vi "Test Start.vi"(11 "Error in":errorcluster) -> (15 "Error out":errorcluster)   [LabVIEW 2020, in "StopWatchTests.lvlib"]
doc: "This VI is used for validating start button in stopwatch"
uses:
  StopWatchTests.lvlib
  <vilib>/SLL Drona/APIs/Stimulus/ControlValue/SetValueAuto.vi
  <vilib>/SLL Drona/APIs/Assert/AssertControlValue/Equal.vi
  <vilib>/SLL Drona/APIs/Get/GetControlValue/GetControlValueByPathString.vi
  <vilib>/SLL Drona/APIs/Stimulus/VI/CloseVI.vi
  <vilib>/Utility/error.llb/Error Cluster From Error Code.vi
  <vilib>/ErrorRing/Error Ring.xnode
  <vilib>/addons/_JKI Toolkits/Caraya/classes/Test/Test.lvclass
  <vilib>/SLL Drona/Drona.lvlib
  <vilib>/SLL Drona/APIs/Stimulus/ControlValue/ControlValue.lvlib
  <vilib>/SLL Drona/APIs/Assert/AssertControlValue/AssertControlValue.lvlib
  <vilib>/SLL Drona/APIs/Get/GetControlValue/GetControlValue.lvlib
  <vilib>/SLL Drona/APIs/Stimulus/VI/VI.lvlib
  <vilib>/Wiresmith Technology/G CLI/CLI Class/CLI.lvclass
panel:
  # "START TEST"
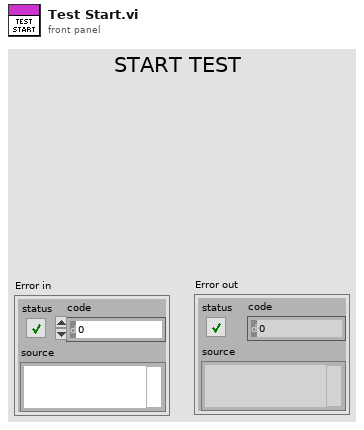
[diagram p1: front panel]
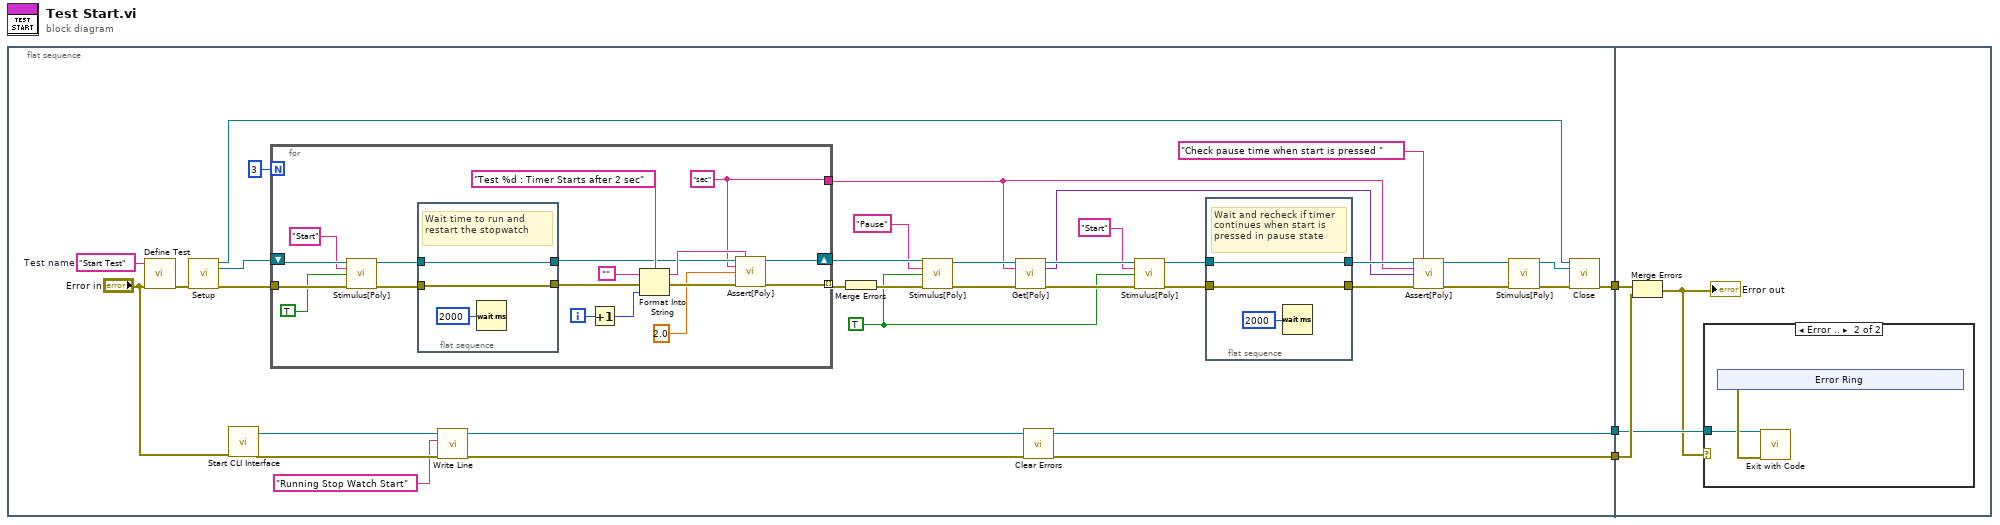
[diagram p0: block diagram]
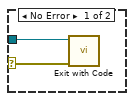
[diagram p2: hidden frame]
diagram:
  n1 = flat-sequence {
    tunnel: [w37] -> w3
    tunnel: [w5] -> w2
    tunnel: [w6] -> w1
    tunnel: w3 -> [w66]
    tunnel: w2 -> [w65]
    tunnel: w1 -> [w64]
    frame #0 {
      w21 = TRUE
      w38 = "Start Test"  # Test name
      n2 = call <vilib>:"Define Test.vi"("error in (no error)"="Error in", "Label (VI Title)"=w38) -> ("error out"=w11:errorcluster)  [unwired: 9 in]
      n3 = call <vilib>:"Setup.vi"("error in"=w11) -> ("Application Ref"=w36:refnum<vi>, "VI Reference Out"=w31:refnum<vi>, "error out"=w32:errorcluster)  [unwired: 12 in]
      n4 = call <vilib>:"Start CLI Interface.vi"("error in (no error)"="Error in") -> ("error out"=w10:errorcluster, "CLI out"=w9:refnum<class "CLI.lvclass">)  [unwired: 7 in, 2 out]
      n5 = for {
        N: 3 -> [_]
        tunnel: w32 -> [w59]
        tunnel: [w44] -> w30 mode=indexing
        shift-right: [w43] -> w27
        shift-left: w31 -> [w58]
        tunnel: [w42] -> w12
        i -> [w49]
        w42 = "sec" ("Control Path")
        n6 = call-poly <vilib>:"Stimulus[Poly].vi"("VI Reference In"=w58, "Control Path"="Start", "Value (Signaling)"=TRUE, "error in"=w59) -> ("VI Reference Out"=w54:refnum<vi>, "error out"=w55:errorcluster)  [unwired: 10 in]
        n7 = flat-sequence {
          tunnel: w55 -> [w61]
          tunnel: [w61] -> w53
          tunnel: w54 -> [w60]
          tunnel: [w60] -> w46
          frame #0 {
            # "Wait time to run and restart the stopwatch"
            n8 = Wait (ms)(milliseconds to wait=u32 2000) -> ()  [unwired: 1 out]
          }
        }
        n9 = Increment(x=w49) -> (x+1=w48:i32)
        n10 = Format Into String(format string="Test %d : Timer Starts after 2 sec", initial string="", error in=w53, w48) -> (resulting string=w47:string, error out=w52:errorcluster)
        n11 = call-poly <vilib>:"Assert[Poly].vi"("VI Reference In"=w46, "Test Label"=w47, "Control Path"=w42, "Control Value"=2.0, "Error In"=w52) -> ("VI Reference Out"=w43:refnum<vi>, "Error Out"=w44:errorcluster)  [unwired: 9 in]
      }
      n12 = call <vilib>:"Write Line.vi"("error in (no error)"=w10, "Text to Write"="Running Stop Watch Start", "CLI in"=w9) -> ("error out"=w7:errorcluster, "CLI out"=w6:refnum<class "CLI.lvclass">)  [unwired: 7 in]
      n13 = Merge Errors(w30) -> (w29:errorcluster)
      n14 = call-poly <vilib>:"Stimulus[Poly].vi"("VI Reference In"=w27, "Control Path"="Pause", "Value (Signaling)"=w21, "error in"=w29) -> ("VI Reference Out"=w24:refnum<vi>, "error out"=w28:errorcluster)  [unwired: 10 in]
      n15 = call-poly <vilib>:"Get[Poly].vi"("VI Reference In"=w24, "Control Path"=w12, "error in"=w28) -> ("VI Reference Out"=w23:refnum<vi>, "Value"=w15:variant, "error out"=w25:errorcluster)  [unwired: 10 in]
      n16 = call <vilib>:"Clear Errors.vi"("error in (no error)"=w7) -> ("error out"=w5:errorcluster)  [unwired: 5 in, 1 out]
      n17 = call-poly <vilib>:"Stimulus[Poly].vi"("VI Reference In"=w23, "Control Path"="Start", "Value (Signaling)"=w21, "error in"=w25) -> ("VI Reference Out"=w19:refnum<vi>, "error out"=w20:errorcluster)  [unwired: 10 in]
      n18 = flat-sequence {
        tunnel: [w40] -> w18
        tunnel: w20 -> [w40]
        tunnel: w19 -> [w39]
        tunnel: [w39] -> w16
        frame #0 {
          # "Wait and recheck if timer continues when start is pressed in pause state"
          n19 = Wait (ms)(milliseconds to wait=u32 2000) -> ()  [unwired: 1 out]
        }
      }
      n20 = call-poly <vilib>:"Assert[Poly].vi"("VI Reference In"=w16, "Test Label"="Check pause time when start is pressed ", "Control Path"=w12, "Control Value"=w15, "Error In"=w18) -> ("VI Reference Out"=w13:refnum<vi>, "Error Out"=w17:errorcluster)  [unwired: 9 in]
      n21 = call-poly <vilib>:"Stimulus[Poly].vi"("VI Reference In"=w13, "error in"=w17) -> ("VI Reference Out"=w35:refnum<vi>, "error out"=w34:errorcluster)  [unwired: 12 in]
      n22 = call <vilib>:"Close.vi"("Application Ref"=w36, "VI Reference"=w35, "error in"=w34) -> ("error out"=w37:errorcluster)  [unwired: 12 in]
    }
    frame #1 {
      n23 = Merge Errors(w66, w65) -> (w63:errorcluster)
      "Error out" <- w63
      n24 = case shown="Error .." w63 {
        selector: w63 -> [w68 _]
        tunnel: w64 -> [w67 w69]
        frame No Error {
          n25 = call <vilib>:"Exit with Code.vi"("error in (no error)"=w68, "CLI in"=w67) -> ()  [unwired: 9 in, 1 out]
        }
        frame Error {
          n26 = xnode "Error Ring"() -> ("error out"=w70:errorcluster)
          n27 = call <vilib>:"Exit with Code.vi"("error in (no error)"=w70, "CLI in"=w69) -> ()  [unwired: 9 in, 1 out]
        }
      }
    }
  }
